vi "Testing_Printer.vi"() -> ()   [LabVIEW 2017]
uses:
  2b9a1f4a-5240-4696-b8f1-e2ace7827ddc.vi
  799b1b0d-2d37-49bd-9ebf-8c413fa797b7.vi
panel:
  in  "remote port or service name":u16
  in  "Start Print":bool
  in  "Printer IP Address":string
  in  "PRN FIle brows":path=path "C:/Users/Aseem/Downloads/TATA123.prn"
  in  "read prn file":bool
  out "error in (no error)":errorcluster
  in  "stop":bool
  out "text":string
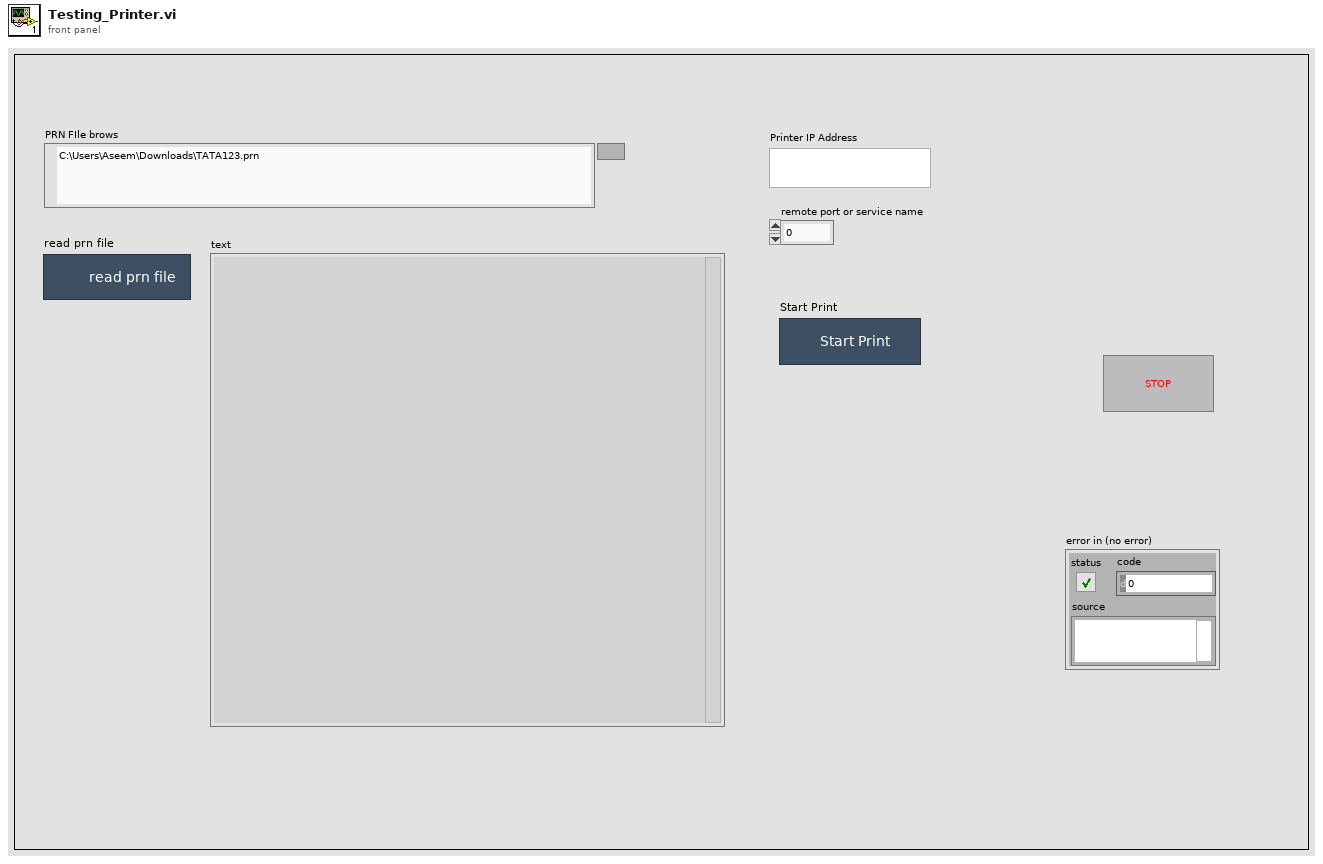
[diagram p1: front panel]
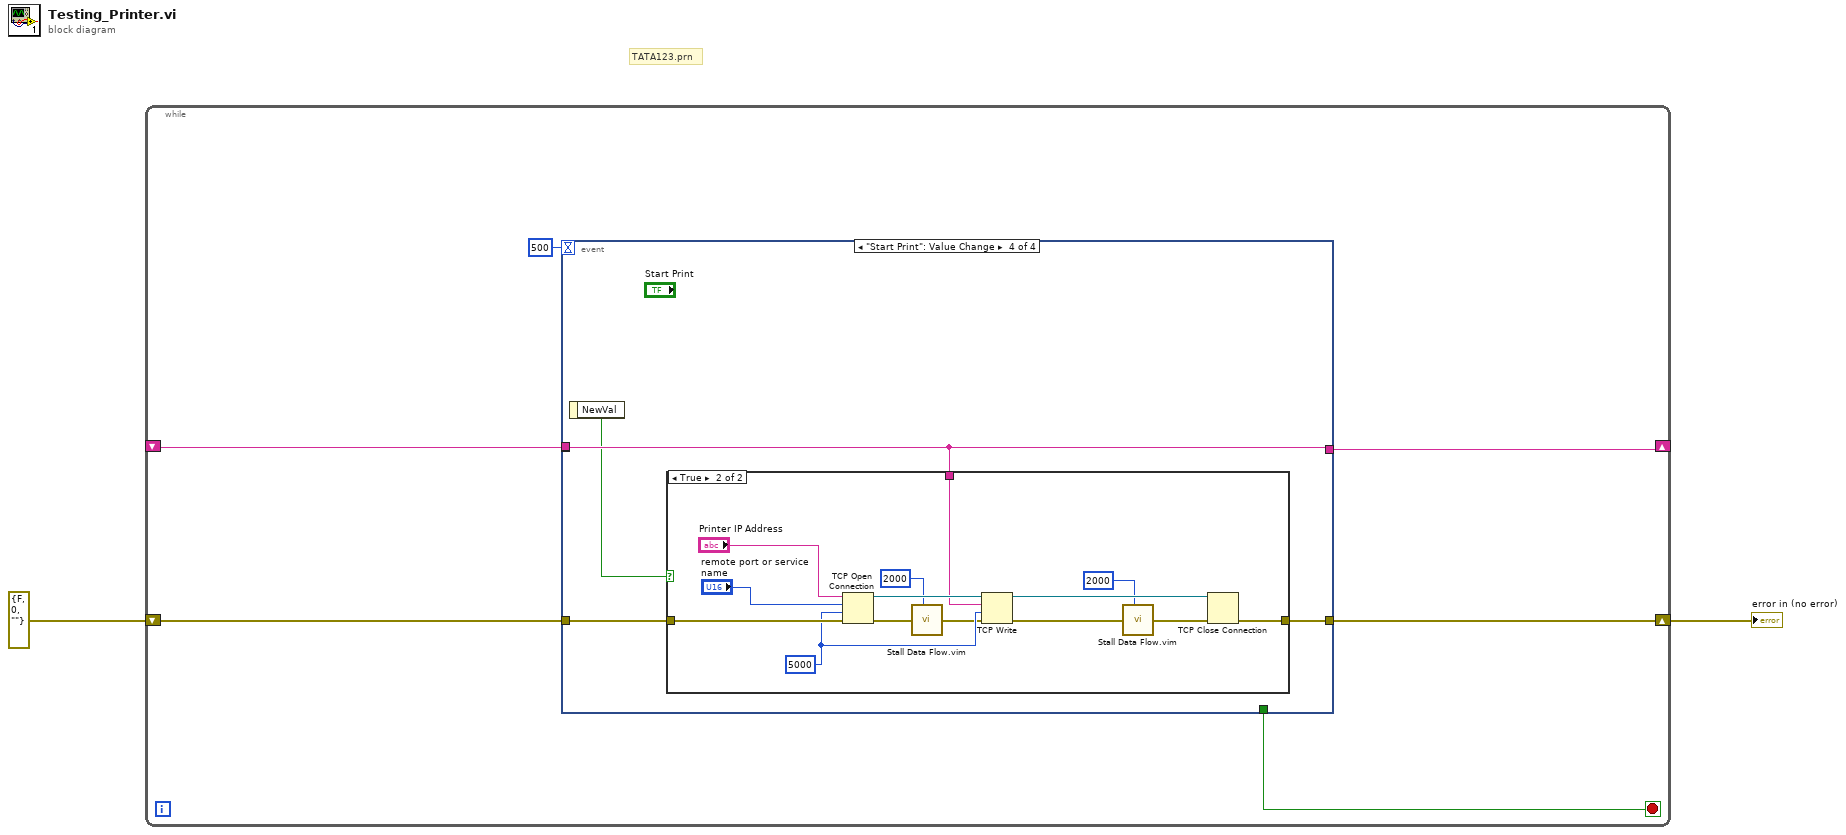
[diagram p0: block diagram]
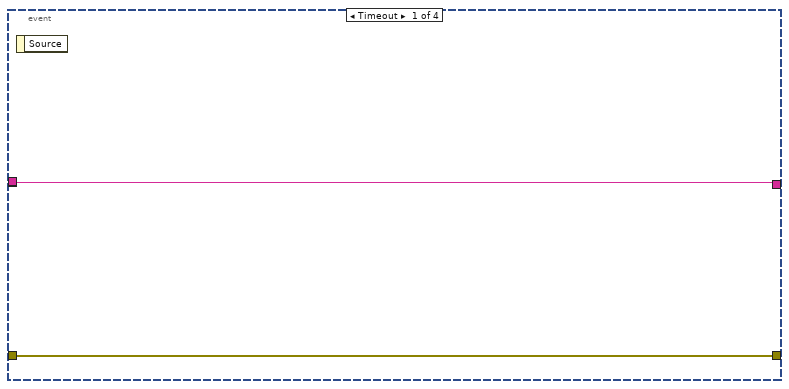
[diagram p2: hidden frame]
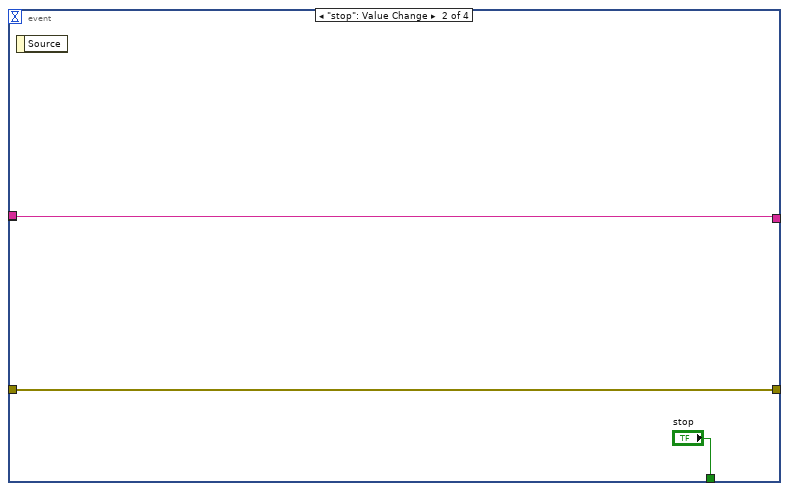
[diagram p3: hidden frame]
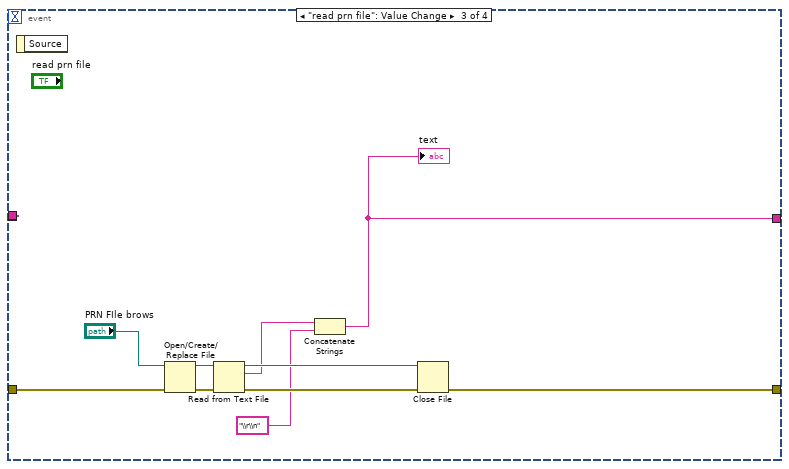
[diagram p4: hidden frame]
diagram:
  # "TATA123.prn"
  n1 = while {
    shift-right: [w8] -> w1
    shift-left: errorcluster {"status"=FALSE, "code"=0, "source"=""} ("error in (no error)") -> [w7]
    shift-right: [w4] -> _
    shift-left: _ -> [w3]
    stop <- w6 stop-if-true
    n2 = event shown="[3] \"Start Print\": Value Change" {
      selector: _ -> [_ _ _ _]
      dyn-events: _ -> [_ _ _ _]
      timeout: 500 -> [_ _ _ _]
      tunnel: [w10 w12 w18 w28] -> w8
      tunnel: w7 -> [w10 w12 w19 w27]
      tunnel: [_ "stop" _ _] -> w6
      tunnel: [w9 w11 w14 w26] -> w4
      tunnel: w3 -> [w9 w11 w17 w26]
      tunnel: [_ _ w17 _] -> _
      event Timeout {
        n3 = event-data() -> ()  [unwired: 1 in, 1 out]
      }
      event "stop": Value Change {
        n4 = event-data() -> ()  [unwired: 1 in, 1 out]
      }
      event "read prn file": Value Change {
        n5 = event-data() -> ()  [unwired: 1 in, 1 out]
        n6 = Open/Create/Replace File(file path (use dialog)="PRN FIle brows", error in=w19) -> (refnum out=w23:refnum<file>, error out=w21:errorcluster)  [unwired: 4 in, 1 out]
        n7 = Read from Text File(file (use dialog)=w23, error in=w21) -> (refnum out=w24:refnum<file>, text=w15:string, error out=w20:errorcluster)  [unwired: 2 in, 1 out]
        n8 = Concatenate Strings(w15, "\\r\\n") -> (w14:string)
        "text" <- w14
        n9 = Close File(refnum=w24, error in=w20) -> (error out=w18:errorcluster)  [unwired: 1 out]
      }
      event "Start Print": Value Change {
        n10 = event-data() -> ("NewVal"=w25:bool)  [unwired: 1 in]
        n11 = case shown="True" w25 {
          tunnel: [w29 w43] -> w28
          tunnel: w27 -> [w29 w38]
          tunnel: w26 -> [_ w30]
          frame False {
          }
          frame True {
            w35 = 5000 ("timeout ms (60000)")
            n12 = TCP Open Connection(address="Printer IP Address", remote port or service name="remote port or service name", timeout ms (60000)=w35, error in (no error)=w38) -> (connection ID=w41:refnum<k5>, error out=w40:errorcluster)  [unwired: 1 in]
            n13 = call "Stall Data Flow.vim"("value in"=w40, "milliseconds to wait"=u32 2000) -> ("value out"=w34:errorcluster)  [unwired: 1 out]
            n14 = TCP Write(connection ID=w41, data in=w30, error in (no error)=w34, 9:w35) -> (connection ID out=w39:refnum<k5>, error out=w42:errorcluster)  [unwired: 1 out]
            n15 = call "Stall Data Flow.vim"("value in"=w42, "milliseconds to wait"=u32 2000) -> ("value out"=w32:errorcluster)  [unwired: 1 out]
            n16 = TCP Close Connection(connection ID=w39, error in (no error)=w32) -> (error out=w43:errorcluster)  [unwired: 2 out]
          }
        }
      }
    }
  }
  "error in (no error)" <- w1
